vi "pmu_Find Phasor Indexes.vi"(6 "physical channel in":T5(array[cluster]), 7 "phasor names":string[](array[string]), 8 "error in (no error)":errorcluster, 9 "3-phase system IDs":u8[](array[numeric]), 10 "phasor phases":T1(array[ring]), 11 "phasor units":u32[](array[numeric])) -> (0 "error out":errorcluster, 3 "phasor channel info":T2[](array[typedef]))   [LabVIEW 2014, in "NI_EP_PMU.lvlib"]
uses:
  <vilib>/addons/Electrical Power/PMU/NI_EP_PMU.lvlib
  <vilib>/addons/Electrical Power/PMU/Common/Controls/pmu_Channel Phase.ctl
  <vilib>/addons/Electrical Power/PMU/Common/Controls/pmu_Phasor Channel Info.ctl
  <vilib>/addons/Electrical Power/PMU/Common/Controls/pmu_Connection Type.ctl
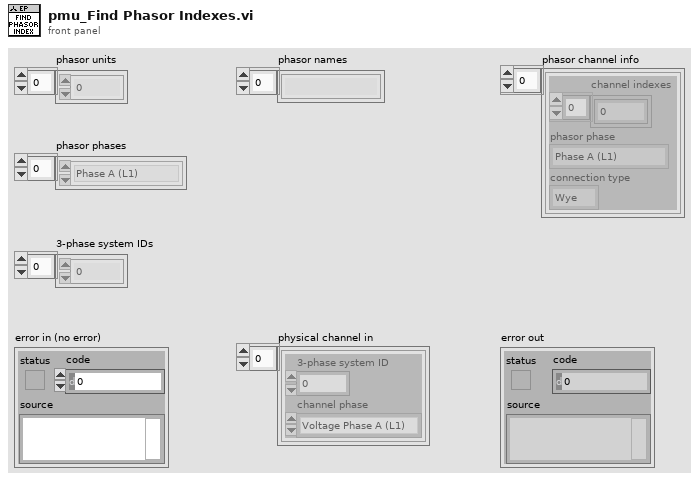
[diagram p1: front panel]
types:
  T1 = enum16{"Phase A (L1)", "Phase B (L2)", "Phase C (L3)", "Phase N", "Positive sequence", "Negative sequence", "Zero sequence"}[]
  T2 = typedef "NI_EP_PMU.lvlib/pmu_Phasor Channel Info.ctl" = cluster{"channel indexes":i32[], "phasor phase":enum16{"Phase A (L1)", "Phase B (L2)", "Phase C (L3)", "Phase N", "Positive sequence", "Negative sequence", "Zero sequence"}, "connection type":T3}
  T3 = typedef "NI_EP_PMU.lvlib/pmu_Connection Type.ctl" = enum16{"Wye", "Delta"}
  T4 = typedef "NI_EP_PMU.lvlib/pmu_Channel Phase.ctl" = enum16{"Voltage Phase A (L1)", "Voltage Phase B (L2)", "Voltage Phase C (L3)", "Voltage Phase N (Neutral)", "Current Phase A (L1)", "Current Phase B (L2)", "Current Phase C (L3)", "Current Phase N (Neutral)", "Voltage Phase AB (L1L2)", "Voltage Phase BC (L2L3)", "Voltage Phase CA (L3L1)"}
  T5 = cluster{"3-phase system ID":u8, "channel phase":T4}[]
  T6 = cluster{"3-phase system ID":u8, "channel phase":T4}
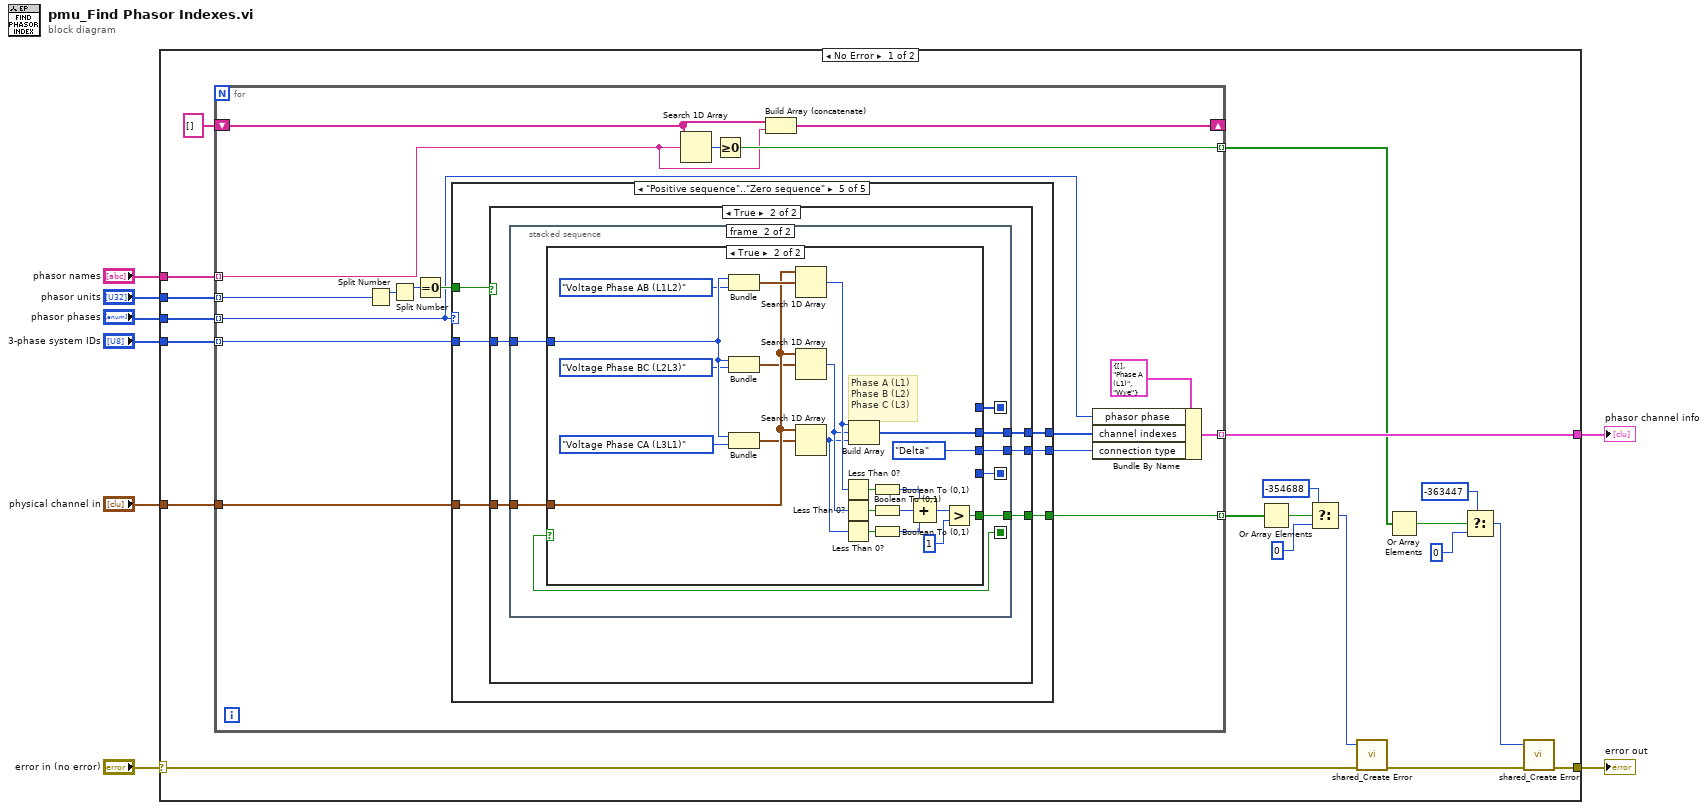
[diagram p0: block diagram]
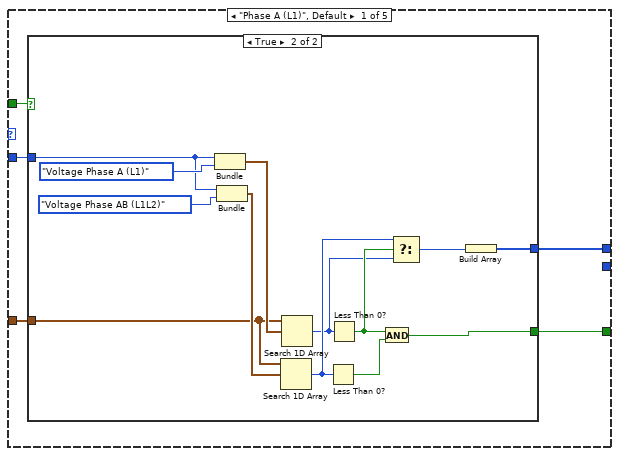
[diagram p2: hidden frame]
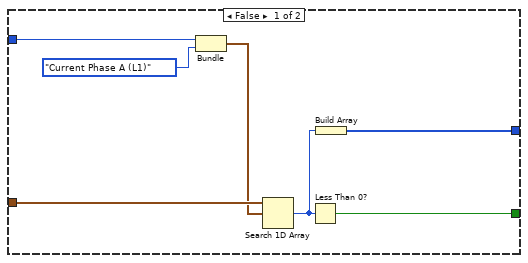
[diagram p3: hidden frame]
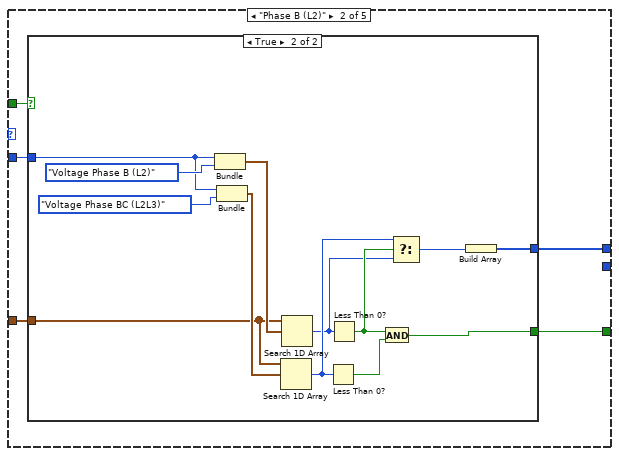
[diagram p4: hidden frame]
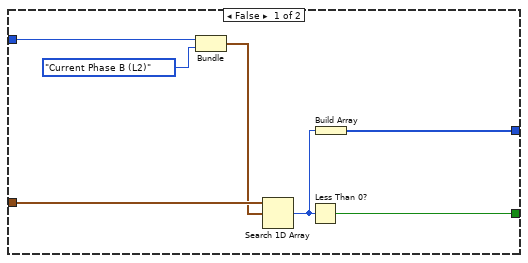
[diagram p5: hidden frame]
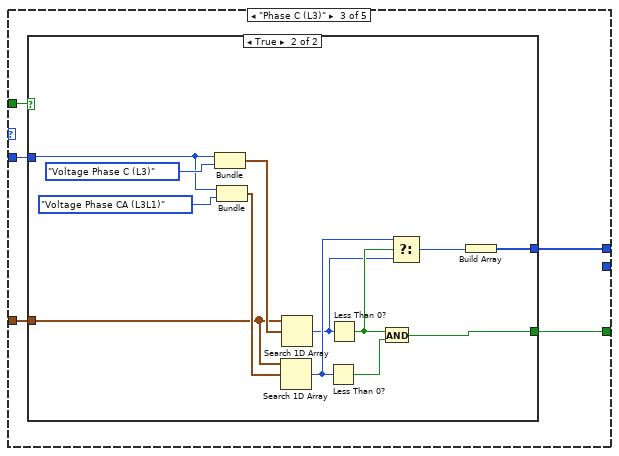
[diagram p6: hidden frame]
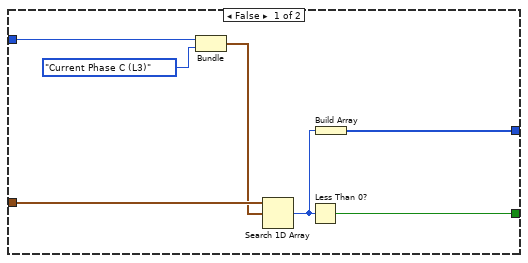
[diagram p7: hidden frame]
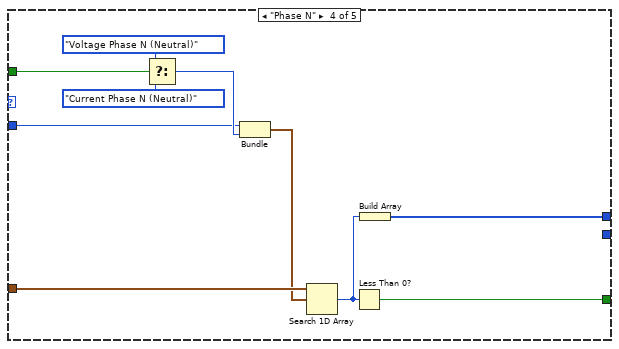
[diagram p8: hidden frame]
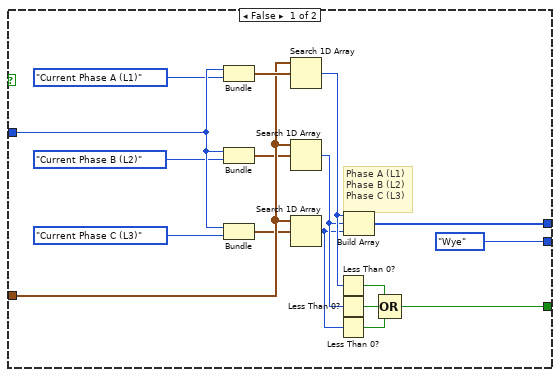
[diagram p9: hidden frame]
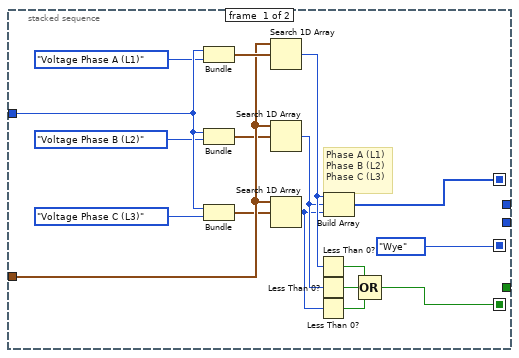
[diagram p10: hidden frame]
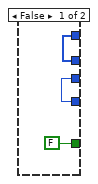
[diagram p11: hidden frame]
diagram:
  n1 = case shown="No Error" "error in (no error)" {
    selector: "error in (no error)" -> [w22 w209]
    tunnel: "physical channel in" -> [w21 _]
    tunnel: [w13 w209] -> w6
    tunnel: [w26 _] -> w5
    tunnel: "phasor names" -> [w12 _]
    tunnel: "phasor units" -> [w11 _]
    tunnel: "phasor phases" -> [w10 _]
    tunnel: "3-phase system IDs" -> [w9 _]
    frame No Error {
      n2 = for {
        tunnel: w21 -> [w42]
        tunnel: [w41] -> w28 mode=indexing
        tunnel: [w40] -> w26 mode=indexing
        shift-right: [w34] -> _
        shift-left: string[] [] -> [w35]
        tunnel: [w33] -> w19 mode=indexing
        tunnel: w12 -> [w32] mode=indexing
        tunnel: w11 -> [w31] mode=indexing
        tunnel: w10 -> [w30] mode=indexing
        tunnel: w9 -> [w29] mode=indexing
        n3 = Split Number(x=w31) -> (hi(x)=w45:u16)  [unwired: 1 out]
        n4 = Split Number(x=w45) -> (hi(x)=w44:u8)  [unwired: 1 out]
        n5 = Equal To 0?(x=w44) -> (x = 0?=w43:bool)
        n6 = case shown="\"Positive sequence\"..\"Zero sequence\"" w30 {
          tunnel: w29 -> [w50 w75 w100 w126 w136]
          tunnel: w43 -> [w46 w71 w96 w128 w132]
          tunnel: w42 -> [w49 w74 w99 w125 w135]
          tunnel: [w48 w73 w98 w124 w134] -> w41
          tunnel: [w47 w72 w97 w122 w133] -> w38
          tunnel: [_ _ _ _ w131] -> w37
          frame "Phase A (L1)", Default {
            n7 = case shown="True" w46 {
              tunnel: w50 -> [w57 w67]
              tunnel: w49 -> [w56 w64]
              tunnel: [w55 w63] -> w48
              tunnel: [w53 w69] -> w47
              frame False {
                n8 = Bundle("3-phase system ID"=w57, "channel phase"=pmu_Channel_Phase."Current Phase A (L1)") -> (w54:T6)  [unwired: 1 in]
                n9 = Search 1D Array(1D array=w56, element=w54) -> (index of element=w52:i32)  [unwired: 1 in]
                n10 = Less Than 0?(x=w52) -> (x < 0?=w55:bool)
                n11 = Build Array(w52) -> (w53:i32[])
              }
              frame True {
                n12 = Bundle("3-phase system ID"=w67, "channel phase"=pmu_Channel_Phase."Voltage Phase A (L1)") -> (w70:T6)  [unwired: 1 in]
                n13 = Bundle("3-phase system ID"=w67, "channel phase"=pmu_Channel_Phase."Voltage Phase AB (L1L2)") -> (w65:T6)  [unwired: 1 in]
                n14 = Search 1D Array(1D array=w64, element=w65) -> (index of element=w60:i32)  [unwired: 1 in]
                n15 = Search 1D Array(1D array=w64, element=w70) -> (index of element=w59:i32)  [unwired: 1 in]
                n16 = Less Than 0?(x=w60) -> (x < 0?=w62:bool)
                n17 = Less Than 0?(x=w59) -> (x < 0?=w61:bool)
                n18 = And(x=w61, y=w62) -> (x .and. y?=w63:bool)
                n19 = Select(t=w60, s=w61, f=w59) -> (s? t:f=w58:i32)
                n20 = Build Array(w58) -> (w69:i32[])
              }
            }
          }
          frame "Phase B (L2)" {
            n21 = case shown="True" w71 {
              tunnel: w75 -> [w82 w92]
              tunnel: w74 -> [w81 w89]
              tunnel: [w80 w88] -> w73
              tunnel: [w78 w94] -> w72
              frame False {
                n22 = Bundle("3-phase system ID"=w82, "channel phase"=pmu_Channel_Phase."Current Phase B (L2)") -> (w79:T6)  [unwired: 1 in]
                n23 = Search 1D Array(1D array=w81, element=w79) -> (index of element=w77:i32)  [unwired: 1 in]
                n24 = Less Than 0?(x=w77) -> (x < 0?=w80:bool)
                n25 = Build Array(w77) -> (w78:i32[])
              }
              frame True {
                n26 = Bundle("3-phase system ID"=w92, "channel phase"=pmu_Channel_Phase."Voltage Phase B (L2)") -> (w95:T6)  [unwired: 1 in]
                n27 = Bundle("3-phase system ID"=w92, "channel phase"=pmu_Channel_Phase."Voltage Phase BC (L2L3)") -> (w90:T6)  [unwired: 1 in]
                n28 = Search 1D Array(1D array=w89, element=w90) -> (index of element=w85:i32)  [unwired: 1 in]
                n29 = Search 1D Array(1D array=w89, element=w95) -> (index of element=w84:i32)  [unwired: 1 in]
                n30 = Less Than 0?(x=w85) -> (x < 0?=w87:bool)
                n31 = Less Than 0?(x=w84) -> (x < 0?=w86:bool)
                n32 = And(x=w86, y=w87) -> (x .and. y?=w88:bool)
                n33 = Select(t=w85, s=w86, f=w84) -> (s? t:f=w83:i32)
                n34 = Build Array(w83) -> (w94:i32[])
              }
            }
          }
          frame "Phase C (L3)" {
            n35 = case shown="True" w96 {
              tunnel: w100 -> [w107 w117]
              tunnel: w99 -> [w106 w114]
              tunnel: [w105 w113] -> w98
              tunnel: [w103 w119] -> w97
              frame False {
                n36 = Bundle("3-phase system ID"=w107, "channel phase"=pmu_Channel_Phase."Current Phase C (L3)") -> (w104:T6)  [unwired: 1 in]
                n37 = Search 1D Array(1D array=w106, element=w104) -> (index of element=w102:i32)  [unwired: 1 in]
                n38 = Less Than 0?(x=w102) -> (x < 0?=w105:bool)
                n39 = Build Array(w102) -> (w103:i32[])
              }
              frame True {
                n40 = Bundle("3-phase system ID"=w117, "channel phase"=pmu_Channel_Phase."Voltage Phase C (L3)") -> (w120:T6)  [unwired: 1 in]
                n41 = Bundle("3-phase system ID"=w117, "channel phase"=pmu_Channel_Phase."Voltage Phase CA (L3L1)") -> (w115:T6)  [unwired: 1 in]
                n42 = Search 1D Array(1D array=w114, element=w115) -> (index of element=w110:i32)  [unwired: 1 in]
                n43 = Search 1D Array(1D array=w114, element=w120) -> (index of element=w109:i32)  [unwired: 1 in]
                n44 = Less Than 0?(x=w110) -> (x < 0?=w112:bool)
                n45 = Less Than 0?(x=w109) -> (x < 0?=w111:bool)
                n46 = And(x=w111, y=w112) -> (x .and. y?=w113:bool)
                n47 = Select(t=w110, s=w111, f=w109) -> (s? t:f=w108:i32)
                n48 = Build Array(w108) -> (w119:i32[])
              }
            }
          }
          frame "Phase N" {
            n49 = Select(t=pmu_Channel_Phase."Voltage Phase N (Neutral)" ("channel phase"), s=w128, f=pmu_Channel_Phase."Current Phase N (Neutral)" ("channel phase")) -> (s? t:f=w127:T4)
            n50 = Bundle("3-phase system ID"=w126, "channel phase"=w127) -> (w123:T6)  [unwired: 1 in]
            n51 = Search 1D Array(1D array=w125, element=w123) -> (index of element=w121:i32)  [unwired: 1 in]
            n52 = Less Than 0?(x=w121) -> (x < 0?=w124:bool)
            n53 = Build Array(w121) -> (w122:i32[])
          }
          frame "Positive sequence".."Zero sequence" {
            n54 = case shown="True" w132 {
              tunnel: w136 -> [w152 w158]
              tunnel: w135 -> [w151 w157]
              tunnel: [w147 w156] -> w134
              tunnel: [w141 w155] -> w133
              tunnel: [pmu_Connection_Type."Wye" ("connection type") w154] -> w131
              frame False {
                # "Phase A (L1)\nPhase B (L2)\nPhase C (L3)"
                n55 = Bundle("3-phase system ID"=w152, "channel phase"=pmu_Channel_Phase."Current Phase A (L1)") -> (w153:T6)  [unwired: 1 in]
                n56 = Bundle("3-phase system ID"=w152, "channel phase"=pmu_Channel_Phase."Current Phase B (L2)") -> (w149:T6)  [unwired: 1 in]
                n57 = Bundle("3-phase system ID"=w152, "channel phase"=pmu_Channel_Phase."Current Phase C (L3)") -> (w150:T6)  [unwired: 1 in]
                n58 = Search 1D Array(1D array=w151, element=w153) -> (index of element=w144:i32)  [unwired: 1 in]
                n59 = Search 1D Array(1D array=w151, element=w149) -> (index of element=w143:i32)  [unwired: 1 in]
                n60 = Search 1D Array(1D array=w151, element=w150) -> (index of element=w142:i32)  [unwired: 1 in]
                n61 = Less Than 0?(x=w144) -> (x < 0?=w148:bool)
                n62 = Less Than 0?(x=w143) -> (x < 0?=w146:bool)
                n63 = Less Than 0?(x=w142) -> (x < 0?=w145:bool)
                n64 = Build Array(w144, w143, w142) -> (w141:i32[])
                n65 = Compound Arithmetic op=OR(w148, w146, w145) -> (w147:bool)
              }
              frame True {
                n66 = stacked-sequence {
                  seq-local: [w161 _] -> [_ w178]
                  seq-local: [w160 _] -> [_ w177]
                  seq-local: [pmu_Connection_Type."Wye" ("connection type") _] -> [_ w176]
                  tunnel: w158 -> [w174 w183]
                  tunnel: w157 -> [w173 w182]
                  tunnel: [_ w180] -> w156
                  tunnel: [_ w181] -> w155
                  tunnel: [_ w179] -> w154
                  frame #0 {
                    # "Phase A (L1)\nPhase B (L2)\nPhase C (L3)"
                    n67 = Bundle("3-phase system ID"=w174, "channel phase"=pmu_Channel_Phase."Voltage Phase A (L1)") -> (w175:T6)  [unwired: 1 in]
                    n68 = Bundle("3-phase system ID"=w174, "channel phase"=pmu_Channel_Phase."Voltage Phase B (L2)") -> (w171:T6)  [unwired: 1 in]
                    n69 = Bundle("3-phase system ID"=w174, "channel phase"=pmu_Channel_Phase."Voltage Phase C (L3)") -> (w172:T6)  [unwired: 1 in]
                    n70 = Search 1D Array(1D array=w173, element=w175) -> (index of element=w167:i32)  [unwired: 1 in]
                    n71 = Search 1D Array(1D array=w173, element=w171) -> (index of element=w166:i32)  [unwired: 1 in]
                    n72 = Search 1D Array(1D array=w173, element=w172) -> (index of element=w165:i32)  [unwired: 1 in]
                    n73 = Less Than 0?(x=w167) -> (x < 0?=w170:bool)
                    n74 = Less Than 0?(x=w166) -> (x < 0?=w169:bool)
                    n75 = Less Than 0?(x=w165) -> (x < 0?=w168:bool)
                    n76 = Build Array(w167, w166, w165) -> (w160:i32[])
                    n77 = Compound Arithmetic op=OR(w170, w169, w168) -> (w161:bool)
                  }
                  frame #1 {
                    n78 = case shown="True" w178 {
                      tunnel: w183 -> [_ w207]
                      tunnel: w182 -> [_ w206]
                      tunnel: [w186 w197] -> w181
                      tunnel: [FALSE w187] -> w180
                      tunnel: [w185 pmu_Connection_Type."Delta" ("connection type")] -> w179
                      tunnel: w177 -> [w186 _]
                      tunnel: w176 -> [w185 _]
                      frame False {
                      }
                      frame True {
                        # "Phase A (L1)\nPhase B (L2)\nPhase C (L3)"
                        n79 = Bundle("3-phase system ID"=w207, "channel phase"=pmu_Channel_Phase."Voltage Phase AB (L1L2)") -> (w208:T6)  [unwired: 1 in]
                        n80 = Bundle("3-phase system ID"=w207, "channel phase"=pmu_Channel_Phase."Voltage Phase BC (L2L3)") -> (w204:T6)  [unwired: 1 in]
                        n81 = Bundle("3-phase system ID"=w207, "channel phase"=pmu_Channel_Phase."Voltage Phase CA (L3L1)") -> (w205:T6)  [unwired: 1 in]
                        n82 = Search 1D Array(1D array=w206, element=w208) -> (index of element=w200:i32)  [unwired: 1 in]
                        n83 = Search 1D Array(1D array=w206, element=w204) -> (index of element=w199:i32)  [unwired: 1 in]
                        n84 = Search 1D Array(1D array=w206, element=w205) -> (index of element=w198:i32)  [unwired: 1 in]
                        n85 = Less Than 0?(x=w200) -> (x < 0?=w203:bool)
                        n86 = Less Than 0?(x=w199) -> (x < 0?=w202:bool)
                        n87 = Less Than 0?(x=w198) -> (x < 0?=w201:bool)
                        n88 = Build Array(w200, w199, w198) -> (w197:i32[])
                        n89 = Boolean To (0,1)(Boolean=w203) -> (0, 1=w192:i16)
                        n90 = Boolean To (0,1)(Boolean=w202) -> (0, 1=w191:i16)
                        n91 = Boolean To (0,1)(Boolean=w201) -> (0, 1=w190:i16)
                        n92 = Compound Arithmetic op=ADD(w192, w191, w190) -> (w189:i16)
                        n93 = Greater?(x=w189, y=i16 1) -> (0:w187:bool)
                      }
                    }
                  }
                }
              }
            }
          }
        }
        n94 = Search 1D Array(1D array=w35, element=w32) -> (index of element=w36:i32)  [unwired: 1 in]
        n95 = Greater Or Equal To 0?(x=w36) -> (x >= 0?=w33:bool)
        n96 = Build Array (concatenate)(w35, w32) -> (w34:string[])
        n97 = Bundle By Name(cluster=T2 {"channel indexes"=[], "phasor phase"=enum."Phase A (L1)", "connection type"=enum."Wye"} ("phasor index"), "phasor phase"=w30, "channel indexes"=w38, "connection type"=w37) -> (w40:T2)
      }
      n98 = Or Array Elements(Boolean array=w28) -> (logical OR=w27:bool)
      n99 = Select(t=-354688 ("error code (0)"), s=w27, f=0 ("error code (0)")) -> (s? t:f=w23:i32)
      n100 = call <vilib>:"shared_Create Error.vi"("error in (no error)"=w22, "error code (0)"=w23) -> ("error out"=w18:errorcluster)  [unwired: 9 in]
      n101 = Or Array Elements(Boolean array=w19) -> (logical OR=w16:bool)
      n102 = Select(t=-363447 ("error code (0)"), s=w16, f=0 ("error code (0)")) -> (s? t:f=w14:i32)
      n103 = call <vilib>:"shared_Create Error.vi"("error in (no error)"=w18, "error code (0)"=w14) -> ("error out"=w13:errorcluster)  [unwired: 9 in]
    }
    frame Error {
    }
  }
  "error out" <- w6
  "phasor channel info" <- w5
